vi "read header&data.vi"(9 "file path(in)":path) -> (0 "Channame":string, 1 "numchans":i32, 3 "ADD1":i32, 4 "Calibration Factor":sgl[](array[numeric]) format="%.2f", 5 "# scans to display":i32, 6 "# of device":i32, 7 "Channel option for device 1":i32[](array[numeric]), 10 "Field strength":i32[](array[numeric]), 11 "Comment":string, 12 "Data Array":i16[][](array[numeric]), 13 "path(out)":path, 14 "Channame2":string, 15 "numchans 2":i32, 17 "ADD2":i32, 18 "Calibration Factor 2":sgl[](array[numeric]) format="%.2f", 19 "# scans to display 2":i32)   [LabVIEW 2013]
panel:
  out "Waveform Graph":i16[][](graph)
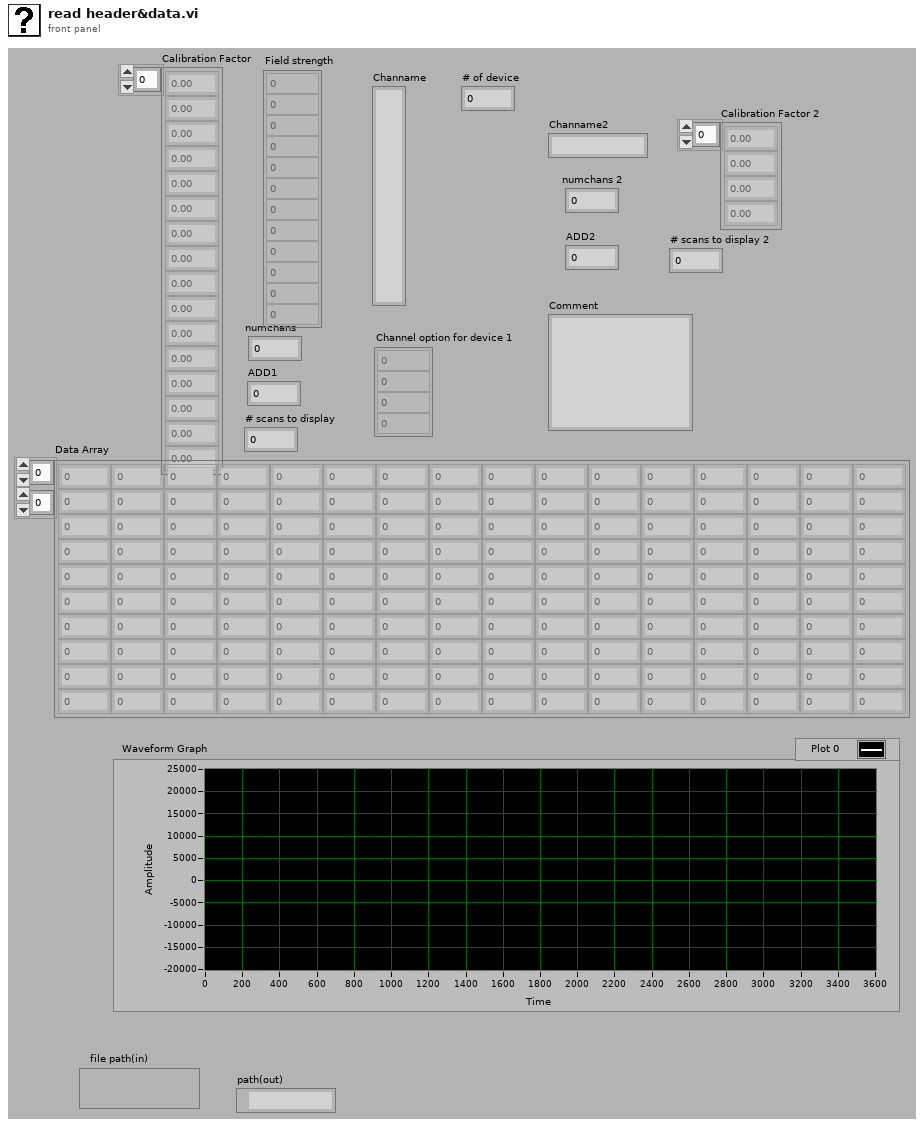
[diagram p1: front panel]
types:
  T1 = enum16{"open", "open or create", "create or replace", "create", "open (read only)"}
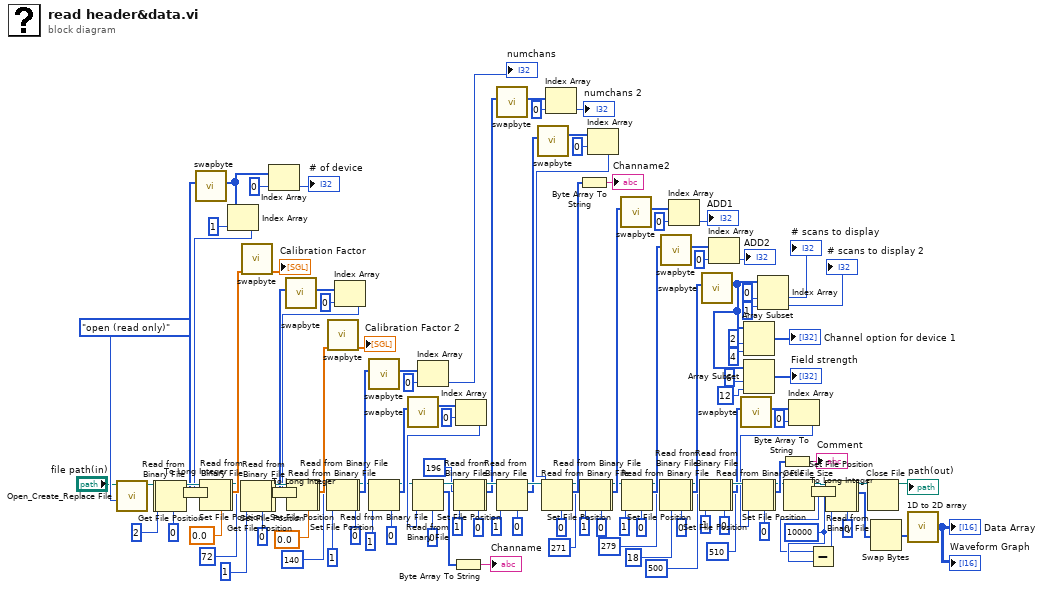
[diagram p0: block diagram]
diagram:
  w32 = 10000 ("pos offset (bytes:0)")
  n1 = call <vilib>:"Open_Create_Replace File.vi"("function (open:0)"=T1."open (read only)", "file path"="file path(in)") -> ("refnum"=w148:refnum<file>)  [unwired: 6 in, 3 out]
  n2 = Read from Binary File(5:0 ("byte stream type"), 10:2 ("count"), 11:w148) -> (0:w2:errorcluster, 2:w127:i32[], 3:w3:refnum<file>)  [unwired: 3 in, 1 out]
  n3 = Get File Position(4:w2, 7:w3) -> (2:w1:i64, 3:w145:refnum<file>)  [unwired: 1 out]
  n4 = To Long Integer(number=w1) -> (32bit integer=w144:i32)
  n5 = call "swapbyte.vi"("I32 1D"=w127) -> ("swapped I32 1D"=w124:i32[])  [unwired: 3 in, 3 out]
  n6 = Set File Position(offset (in bytes) (0)=w144, refnum=w145) -> (refnum out=w5:refnum<file>, error out=w4:errorcluster)  [unwired: 2 in]
  n7 = Index Array(array=w124, index=1 ("Index")) -> (element=w128:i32)
  n8 = Read from Binary File(5:sgl 0.0 ("byte stream type"), 8:w4, 10:w128, 11:w5) -> (2:w142:sgl[], 3:w134:refnum<file>)  [unwired: 2 in, 2 out]
  n9 = Set File Position(offset (in bytes) (0)=72 ("pos offset (0)"), refnum=w134) -> (refnum out=w12:refnum<file>, error out=w11:errorcluster)  [unwired: 2 in]
  n10 = call "swapbyte.vi"("SGL 1D"=w142) -> ("swapped SGL 1D"=→"Calibration Factor":sgl[])  [unwired: 3 in, 3 out]
  n11 = Read from Binary File(5:0 ("byte stream type"), 8:w11, 10:1 ("count"), 11:w12) -> (0:w9:errorcluster, 2:w123:i32[], 3:w10:refnum<file>)  [unwired: 2 in, 1 out]
  n12 = Get File Position(4:w9, 7:w10) -> (2:w8:i64, 3:w135:refnum<file>)  [unwired: 1 out]
  n13 = Index Array(array=w124, index=0 ("Index")) -> (element=→"# of device":i32)
  n14 = To Long Integer(number=w8) -> (32bit integer=w133:i32)
  n15 = call "swapbyte.vi"("I32 1D"=w123) -> ("swapped I32 1D"=w122:i32[])  [unwired: 3 in, 3 out]
  n16 = Set File Position(offset (in bytes) (0)=w133, refnum=w135) -> (refnum out=w7:refnum<file>, error out=w6:errorcluster)  [unwired: 2 in]
  n17 = Index Array(array=w122, index=0 ("Index")) -> (element=w130:i32)
  n18 = Read from Binary File(5:sgl 0.0 ("byte stream type"), 8:w6, 10:w130, 11:w7) -> (2:w140:sgl[], 3:w118:refnum<file>)  [unwired: 2 in, 2 out]
  n19 = Set File Position(offset (in bytes) (0)=140 ("pos offset (0)"), refnum=w118) -> (refnum out=w14:refnum<file>, error out=w13:errorcluster)  [unwired: 2 in]
  n20 = call "swapbyte.vi"("SGL 1D"=w140) -> ("swapped SGL 1D"=→"Calibration Factor 2":sgl[])  [unwired: 3 in, 3 out]
  n21 = Read from Binary File(5:0 ("byte stream type"), 8:w13, 10:1 ("count"), 11:w14) -> (2:w117:i32[], 3:w114:refnum<file>)  [unwired: 2 in, 2 out]
  n22 = call "swapbyte.vi"("I32 1D"=w117) -> ("swapped I32 1D"=w70:i32[])  [unwired: 3 in, 3 out]
  n23 = Read from Binary File(5:0 ("byte stream type"), 10:1 ("count"), 11:w114) -> (2:w113:i32[], 3:w109:refnum<file>)  [unwired: 3 in, 2 out]
  n24 = call "swapbyte.vi"("I32 1D"=w113) -> ("swapped I32 1D"=w112:i32[])  [unwired: 3 in, 3 out]
  n25 = Index Array(array=w70, index=0 ("Index")) -> (element=→"numchans":i32)
  n26 = Index Array(array=w112, index=0 ("Index")) -> (element=w110:i32)
  n27 = Read from Binary File(5:u8 0 ("byte stream type"), 10:w110, 11:w109) -> (2:w107:u8[], 3:w93:refnum<file>)  [unwired: 3 in, 2 out]
  n28 = Byte Array To String(unsigned byte array=w107) -> (string=→"Channame":string)
  n29 = Set File Position(offset (in bytes) (0)=196 ("pos offset (0)"), refnum=w93) -> (refnum out=w16:refnum<file>, error out=w15:errorcluster)  [unwired: 2 in]
  n30 = Read from Binary File(5:0 ("byte stream type"), 8:w15, 10:1 ("count"), 11:w16) -> (2:w95:i32[], 3:w98:refnum<file>)  [unwired: 2 in, 2 out]
  n31 = call "swapbyte.vi"("I32 1D"=w95) -> ("swapped I32 1D"=w73:i32[])  [unwired: 3 in, 3 out]
  n32 = Read from Binary File(5:0 ("byte stream type"), 10:1 ("count"), 11:w98) -> (2:w99:i32[], 3:w103:refnum<file>)  [unwired: 3 in, 2 out]
  n33 = call "swapbyte.vi"("I32 1D"=w99) -> ("swapped I32 1D"=w100:i32[])  [unwired: 3 in, 3 out]
  n34 = Index Array(array=w73, index=0 ("Index")) -> (element=→"numchans 2":i32)
  n35 = Index Array(array=w100, index=0 ("Index")) -> (element=w102:i32)
  n36 = Read from Binary File(5:u8 0 ("byte stream type"), 10:w102, 11:w103) -> (2:w105:u8[], 3:w88:refnum<file>)  [unwired: 3 in, 2 out]
  n37 = Byte Array To String(unsigned byte array=w105) -> (string=→"Channame2":string)
  n38 = Set File Position(offset (in bytes) (0)=271 ("pos offset (0)"), refnum=w88) -> (refnum out=w18:refnum<file>, error out=w17:errorcluster)  [unwired: 2 in]
  n39 = Read from Binary File(5:0 ("byte stream type"), 8:w17, 10:1 ("count"), 11:w18) -> (2:w85:i32[], 3:w76:refnum<file>)  [unwired: 2 in, 2 out]
  n40 = call "swapbyte.vi"("I32 1D"=w85) -> ("swapped I32 1D"=w84:i32[])  [unwired: 3 in, 3 out]
  n41 = Read from Binary File(5:0 ("byte stream type"), 10:1 ("count"), 11:w76) -> (2:w79:i32[], 3:w64:refnum<file>)  [unwired: 3 in, 2 out]
  n42 = Set File Position(offset (in bytes) (0)=279 ("pos offset (0)"), refnum=w64) -> (refnum out=w20:refnum<file>, error out=w19:errorcluster)  [unwired: 2 in]
  n43 = call "swapbyte.vi"("I32 1D"=w79) -> ("swapped I32 1D"=w80:i32[])  [unwired: 3 in, 3 out]
  n44 = Read from Binary File(5:0 ("byte stream type"), 8:w19, 10:18 ("count"), 11:w20) -> (2:w54:i32[], 3:w42:refnum<file>)  [unwired: 2 in, 2 out]
  n45 = Index Array(array=w84, index=0 ("Index")) -> (element=→"ADD1":i32)
  n46 = Set File Position(offset (in bytes) (0)=500 ("pos offset (0)"), refnum=w42) -> (refnum out=w24:refnum<file>, error out=w23:errorcluster)  [unwired: 2 in]
  n47 = call "swapbyte.vi"("I32 1D"=w54) -> ("swapped I32 1D"=w53:i32[])  [unwired: 3 in, 3 out]
  n48 = Read from Binary File(5:0 ("byte stream type"), 8:w23, 10:1 ("count"), 11:w24) -> (2:w50:i32[], 3:w51:refnum<file>)  [unwired: 2 in, 2 out]
  n49 = Index Array(array=w80, index=0 ("Index")) -> (element=→"ADD2":i32)
  n50 = call "swapbyte.vi"("I32 1D"=w50) -> ("swapped I32 1D"=w47:i32[])  [unwired: 3 in, 3 out]
  n51 = Set File Position(offset (in bytes) (0)=510 ("pos offset (0)"), refnum=w51) -> (refnum out=w22:refnum<file>, error out=w21:errorcluster)  [unwired: 2 in]
  n52 = Array Subset(array=w53, index=2 ("Array Index"), length=4 ("Array Length")) -> (→"Channel option for device 1":i32[])
  n53 = Array Subset(array=w53, index=6 ("Array Index"), length=12 ("Array Length")) -> (→"Field strength":i32[])
  n54 = Index Array(array=w53, index #1=0 ("Index"), index #2=1 ("Index")) -> (element #1=→"# scans to display":i32, element #2=→"# scans to display 2":i32)
  n55 = Index Array(array=w47, index=0 ("Index")) -> (element=w45:i32)
  n56 = Read from Binary File(5:u8 0 ("byte stream type"), 8:w21, 10:w45, 11:w22) -> (2:w41:u8[], 3:w35:refnum<file>)  [unwired: 2 in, 2 out]
  n57 = Byte Array To String(unsigned byte array=w41) -> (string=→"Comment":string)
  n58 = Get File Size(file=w35) -> (refnum out=w34:refnum<file>, size (in bytes)=w25:i64)  [unwired: 1 in, 1 out]
  n59 = To Long Integer(number=w25) -> (32bit integer=w31:i32)
  n60 = Subtract(x=w31, y=w32) -> (x-y=w30:i32)
  n61 = Set File Position(offset (in bytes) (0)=w32, refnum=w34) -> (refnum out=w27:refnum<file>, error out=w26:errorcluster)  [unwired: 2 in]
  n62 = Read from Binary File(5:i16 0 ("byte stream type"), 8:w26, 10:w30, 11:w27) -> (2:w33:i16[], 3:w38:refnum<file>)  [unwired: 2 in, 2 out]
  n63 = Close File(refnum=w38) -> (path=→"path(out)":path)  [unwired: 1 in, 1 out]
  n64 = Swap Bytes(anything=w33) -> (byte swapped=w37:i16[])
  n65 = call "1D to 2D array.vi"("1D Array Input"=w37) -> ("2D Array Output"=→"Data Array" →"Waveform Graph":i16[][])  [unwired: 1 in]
